vi "CAlex2_SetAllCuffs_Mobile.vi"(4 "ShankExtraWeight":dbl, 6 "ThighExtraWeight":dbl, 8 "error in (no error)":errorcluster, 10 "LegProperty":T1={"BodyDim"={"ThighLt (m)"=0.4, "ShankLt (m)"=0.41, "HipWd (m)"=0.32}, "BodyWt"={"Thigh (kg)"=0.0, "Shank (kg)"=0.0}, "Cuff Loc"={"HipCuffWd (m)"=0.4, "HipCuffHt (m)"=0.1, "HipFwdShift (m)"=0.0, "ThighToKnee (m)"=0.25, "ThighCuffDist (m)"=0.0, "ShankToKnee (m)"=0.15}}, 11 "CAlex2 in":refnum<class "CAlex2.lvclass">) -> (0 "error out":errorcluster, 3 "CAlex2 out":refnum<class "CAlex2.lvclass">)   [LabVIEW 2016, in "CAlex2.lvclass"]
uses:
  CAlex2.lvclass
  C:/Users/randh/Desktop/CABLE-LABVIEW/CALEX/CAlex2-controller/Classes/SerialChain-Cable/SerialChain-Cable.lvclass
  TypeDef/LowerBodyDim.ctl
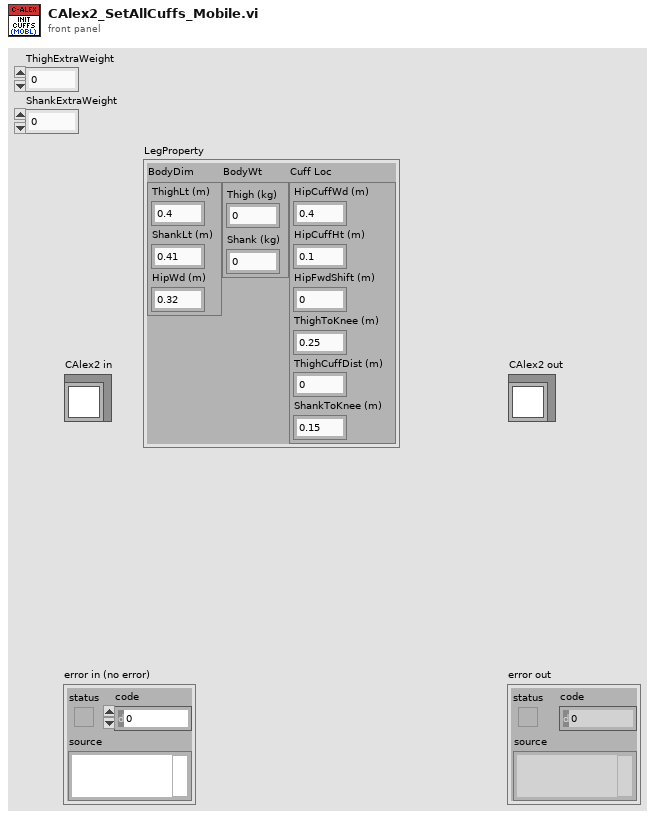
[diagram p1: front panel]
types:
  T1 = typedef "CAlex2.lvclass/LowerBodyDim.ctl" = cluster{"BodyDim":cluster{"ThighLt (m)":dbl, "ShankLt (m)":dbl, "HipWd (m)":dbl}, "BodyWt":cluster{"Thigh (kg)":dbl, "Shank (kg)":dbl}, "Cuff Loc":cluster{"HipCuffWd (m)":dbl, "HipCuffHt (m)":dbl, "HipFwdShift (m)":dbl, "ThighToKnee (m)":dbl, "ThighCuffDist (m)":dbl, "ShankToKnee (m)":dbl}}
  T2 = typedef "SerialChain-Cable.lvclass/Cuff.ctl" = cluster{"BodyID":i32, "CoM(CuffCS)":T3, "Mass(kg)":dbl, "CablePts(CuffCS)":T3[], "Cuff->Body":T4}
  T3 = typedef "SerialChain.lvclass/PointOnBody.ctl" = cluster{"Coord4":dbl[], "ID":i32}
  T4 = typedef "NI_Matrix.lvlib/RealMatrix.ctl" = dbl[][]
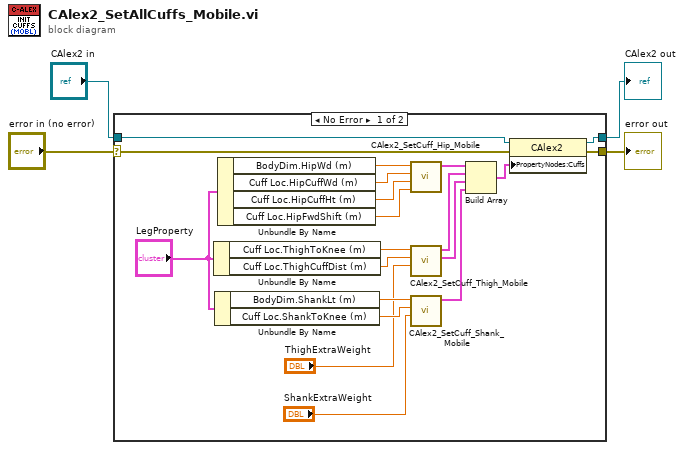
[diagram p0: block diagram]
diagram:
  n1 = case shown="No Error" "error in (no error)" {
    selector: "error in (no error)" -> [w8 w26]
    tunnel: [w22 w26] -> w3
    tunnel: [w23 w25] -> w1
    tunnel: "CAlex2 in" -> [w9 w25]
    frame No Error {
      n2 = Unbundle By Name("LegProperty") -> ("Cuff Loc.ThighToKnee (m)"=w10:dbl, "Cuff Loc.ThighCuffDist (m)"=w5:dbl)
      n3 = Unbundle By Name("LegProperty") -> ("BodyDim.ShankLt (m)"=w17:dbl, "Cuff Loc.ShankToKnee (m)"=w16:dbl)
      n4 = Unbundle By Name("LegProperty") -> ("BodyDim.HipWd (m)"=w14:dbl, "Cuff Loc.HipCuffWd (m)"=w12:dbl, "Cuff Loc.HipCuffHt (m)"=w13:dbl, "Cuff Loc.HipFwdShift (m)"=w11:dbl)
      n5 = call "CAlex2_SetCuff_Hip_Mobile.vi"("Hip Cuff Forward Shift (m)"=w11, "Hip Cuff Height (m)"=w13, "Hip Cuff Width (m)"=w12, "Hip Width (m)"=w14) -> ("Hip Cuff"=w21:T2)  [unwired: 7 in]
      n6 = call "CAlex2_SetCuff_Thigh_Mobile.vi"("Extra Weight (kg)"="ThighExtraWeight", "Upper Cuff to Lower Cuff (m)"=w5, "Lower Cuff to Knee (m)"=w10) -> ("Thigh Cuff Low"=w19:T2, "Thigh Cuff High"=w20:T2)  [unwired: 7 in]
      n7 = call "CAlex2_SetCuff_Shank_Mobile.vi"("ExtraWeight"="ShankExtraWeight", "Distance To Knee"=w16, "Shank Length"=w17) -> ("Shank Cuff"=w18:T2)  [unwired: 8 in]
      n8 = Build Array(w21, w20, w19, w18) -> (w24:T2[])
      n9 = property class="CAlex2"(reference=w9, error in=w8, "PropertyNodes:Cuffs"=w24) -> (reference out=w23:refnum<class "CAlex2.lvclass">, error out=w22:errorcluster)
    }
    frame Error {
    }
  }
  "error out" <- w3
  "CAlex2 out" <- w1
